vi "ex1_snap Color.vi"() -> ()   [LabVIEW 2010]
uses:
  <userlib>/QCam Color Globals.vi
  <userlib>/QI_Transition.llb/QCam Grab Abort.vi
panel:
  in  "SELECT IMAGE TYPE":u16(ring) items=["8 Bit", "16 Bit"]
  out "Images Collected":u64
  in  "Blue Gain":u32=1 min=1 step=1
  in  "Red Gain":u32=1 min=1 step=1
  in  "Green Gain":u32=1 min=1 step=1
  in  "stop":bool
  out "Image":T1(plugin-control)
  in  "Blue Exposure":dbl=483.0
  in  "Red Exposure":dbl=235.0
  in  "Green Exposure":dbl=300.0
  out "error status":errorcluster
  # "msec"
  # "msec"
  # "msec"
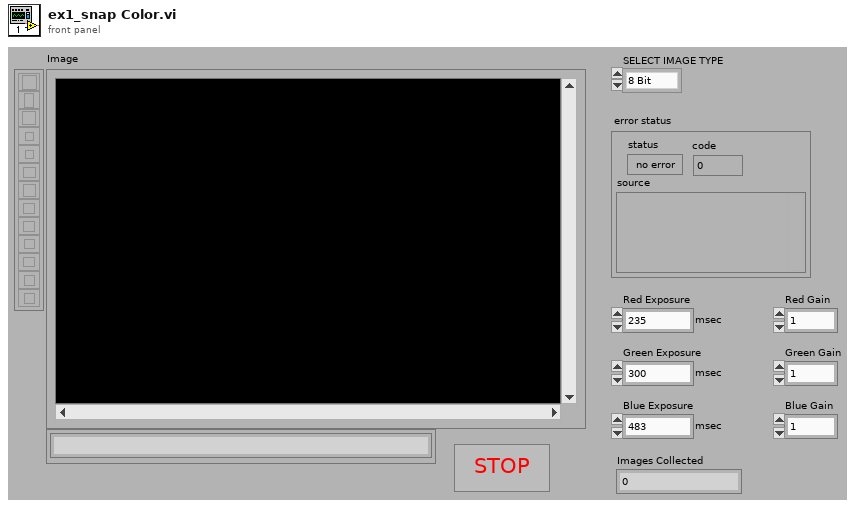
[diagram p1: front panel]
types:
  T1 = typedef "IMAQ Image.ctl" = refnum<image>
  T2 = typedef "Image Type" = u32
  T3 = cluster{"Green Gain":u32, "Red Gain":u32, "Blue Gain":u32}
  T4 = cluster{"Green Exposure":dbl, "Red Exposure":dbl, "Blue Exposure":dbl}
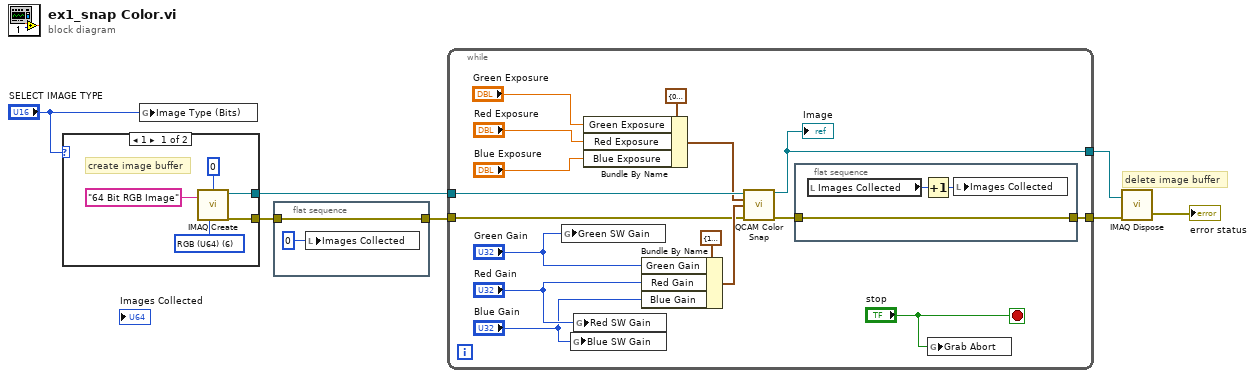
[diagram p0: block diagram]
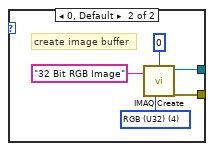
[diagram p2: hidden frame]
diagram:
  # "delete image buffer"
  n1 = case shown="1" "SELECT IMAGE TYPE" {
    tunnel: [w11 w16] -> w7
    tunnel: [w8 w13] -> w3
    frame 1 {
      w9 = T2 6 items=["Grayscale (U8)", "Grayscale (I16)", "Grayscale (SGL)", "Complex (CSG)", "RGB (U32)", "HSL (U32)", "RGB (U64)", "Grayscale (U16)"] ("Image Type")
      # "create image buffer"
      n2 = call "IMAQ Create"("Border Size"=0, "Image Name"="64 Bit RGB Image", "Image Type"=w9) -> ("New Image"=w11:T1, "error out"=w8:errorcluster)  [unwired: 1 in, 1 out]
    }
    frame 0, Default {
      w14 = T2 4 items=["Grayscale (U8)", "Grayscale (I16)", "Grayscale (SGL)", "Complex (CSG)", "RGB (U32)", "HSL (U32)", "RGB (U64)", "Grayscale (U16)"] ("Image Type")
      # "create image buffer"
      n3 = call "IMAQ Create"("Border Size"=0, "Image Name"="32 Bit RGB Image", "Image Type"=w14) -> ("New Image"=w16:T1, "error out"=w13:errorcluster)  [unwired: 1 in, 1 out]
    }
  }
  n4 = global write "QCam Color Globals.vi" "Image Type (Bits)"("SELECT IMAGE TYPE") -> ()
  n5 = flat-sequence {
    tunnel: w3 -> [w18]
    tunnel: [w18] -> w2
    frame #0 {
      n6 = local write "Images Collected"(0) -> ()
    }
  }
  n7 = while {
    tunnel: w7 -> [w35]
    tunnel: w2 -> [w23]
    tunnel: [w29] -> w5
    tunnel: [w24] -> w4
    stop <- "stop" stop-if-true
    n8 = global write "QCam Color Globals.vi" "Green SW Gain"("Green Gain") -> ()
    n9 = global write "QCam Color Globals.vi" "Blue SW Gain"("Blue Gain") -> ()
    n10 = global write "QCam Color Globals.vi" "Red SW Gain"("Red Gain") -> ()
    n11 = Bundle By Name(cluster=T4 {"Green Exposure"=0.0, "Red Exposure"=0.0, "Blue Exposure"=0.0} ("Exposures"), "Green Exposure"="Green Exposure", "Red Exposure"="Red Exposure", "Blue Exposure"="Blue Exposure") -> (w30:T4)
    n12 = Bundle By Name(cluster=T3 {"Green Gain"=1, "Red Gain"=1, "Blue Gain"=1} ("Gains"), "Green Gain"="Green Gain", "Red Gain"="Red Gain", "Blue Gain"="Blue Gain") -> (w27:T3)
    n13 = call <userlib>:"QCAM Color Snap.vi"("New Image"=w35, "Exposures"=w30, "Gains"=w27, "error in (no error)"=w23) -> ("Image Out"=w29:T1, "error out"=w25:errorcluster)  [unwired: 5 in, 5 out]
    "Image" <- w29
    n14 = flat-sequence {
      tunnel: w25 -> [w38]
      tunnel: [w38] -> w24
      frame #0 {
        n15 = local read "Images Collected"() -> (w37:u64)
        n16 = Increment(x=w37) -> (x+1=w36:u64)
        n17 = local write "Images Collected"(w36) -> ()
      }
    }
    n18 = global write "QCam Grab Abort.vi" "Grab Abort"("stop") -> ()
  }
  n19 = call "IMAQ Dispose"("Image"=w5, "error in (no error)"=w4) -> ("error out"=→"error status":errorcluster)  [unwired: 1 in, 3 out]
